vi "运维调试.vi"() -> ()   [LabVIEW 2016]
uses:
  <vilib>/Utility/miscctls.llb/LVPointTypeDef.ctl
  <vilib>/Utility/config.llb/NI_LVConfig.lvlib
panel:
  in  "运维调试菜单":T1
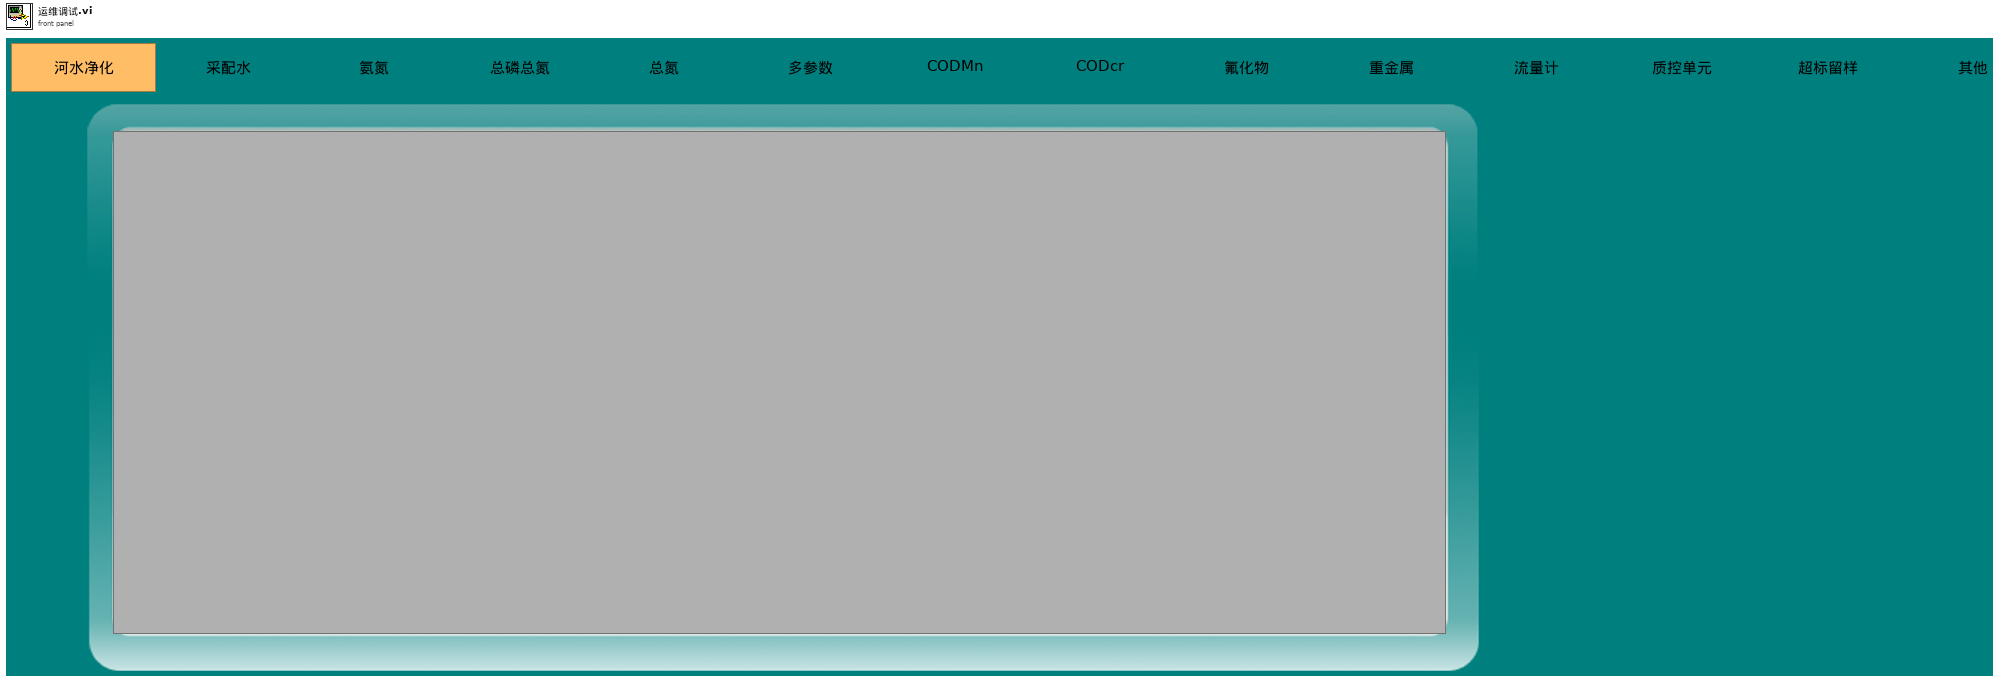
[diagram p1: front panel]
types:
  T1 = typedef "运维调试单选控件.ctl" = enum32{"河水净化", "采配水", "氨氮", "总磷总氮", "总氮", "多参数", "CODMn", "CODcr", "氟化物", "重金属", "流量计", "质控单元", "超标留样", "其他"}
  T2 = typedef "LVPointTypeDef.ctl" = cluster{"Horizontal":i16, "Vertical":i16}
  T3 = typedef "设备类型.ctl" = enum16{"微站", "固定站", "浮船"}
  T4 = typedef "采配水类型.ctl" = enum16{"V1", "V2", "V3", "V4", "室内V1", "室内V2", "固定站V1", "固定站V2", "浮船V1", "浮船V2"}
  T5 = typedef "氨氮总磷总氮模块版本.ctl" = enum16{"V2", "V3"}
  T6 = typedef "多参数模块版本.ctl" = enum16{"原位多参数", "集成式多参"}
  T7 = typedef "CODMn模块版本.ctl" = enum16{"PLC版", "单片机版", "通用流路版本"}
  T8 = typedef "CODcr模块版本.ctl" = enum16{"斯坦道V3", "点创"}
  T9 = typedef "加标回收模块版本.ctl" = enum16{"V1", "V2", "V4"}
  T10 = typedef "NI_LVConfig.lvlib/Config Data RefNum.ctl" = refnum<k1>
  T11 = enum32{"Bad", "Idle", "Run top level", "Running"}
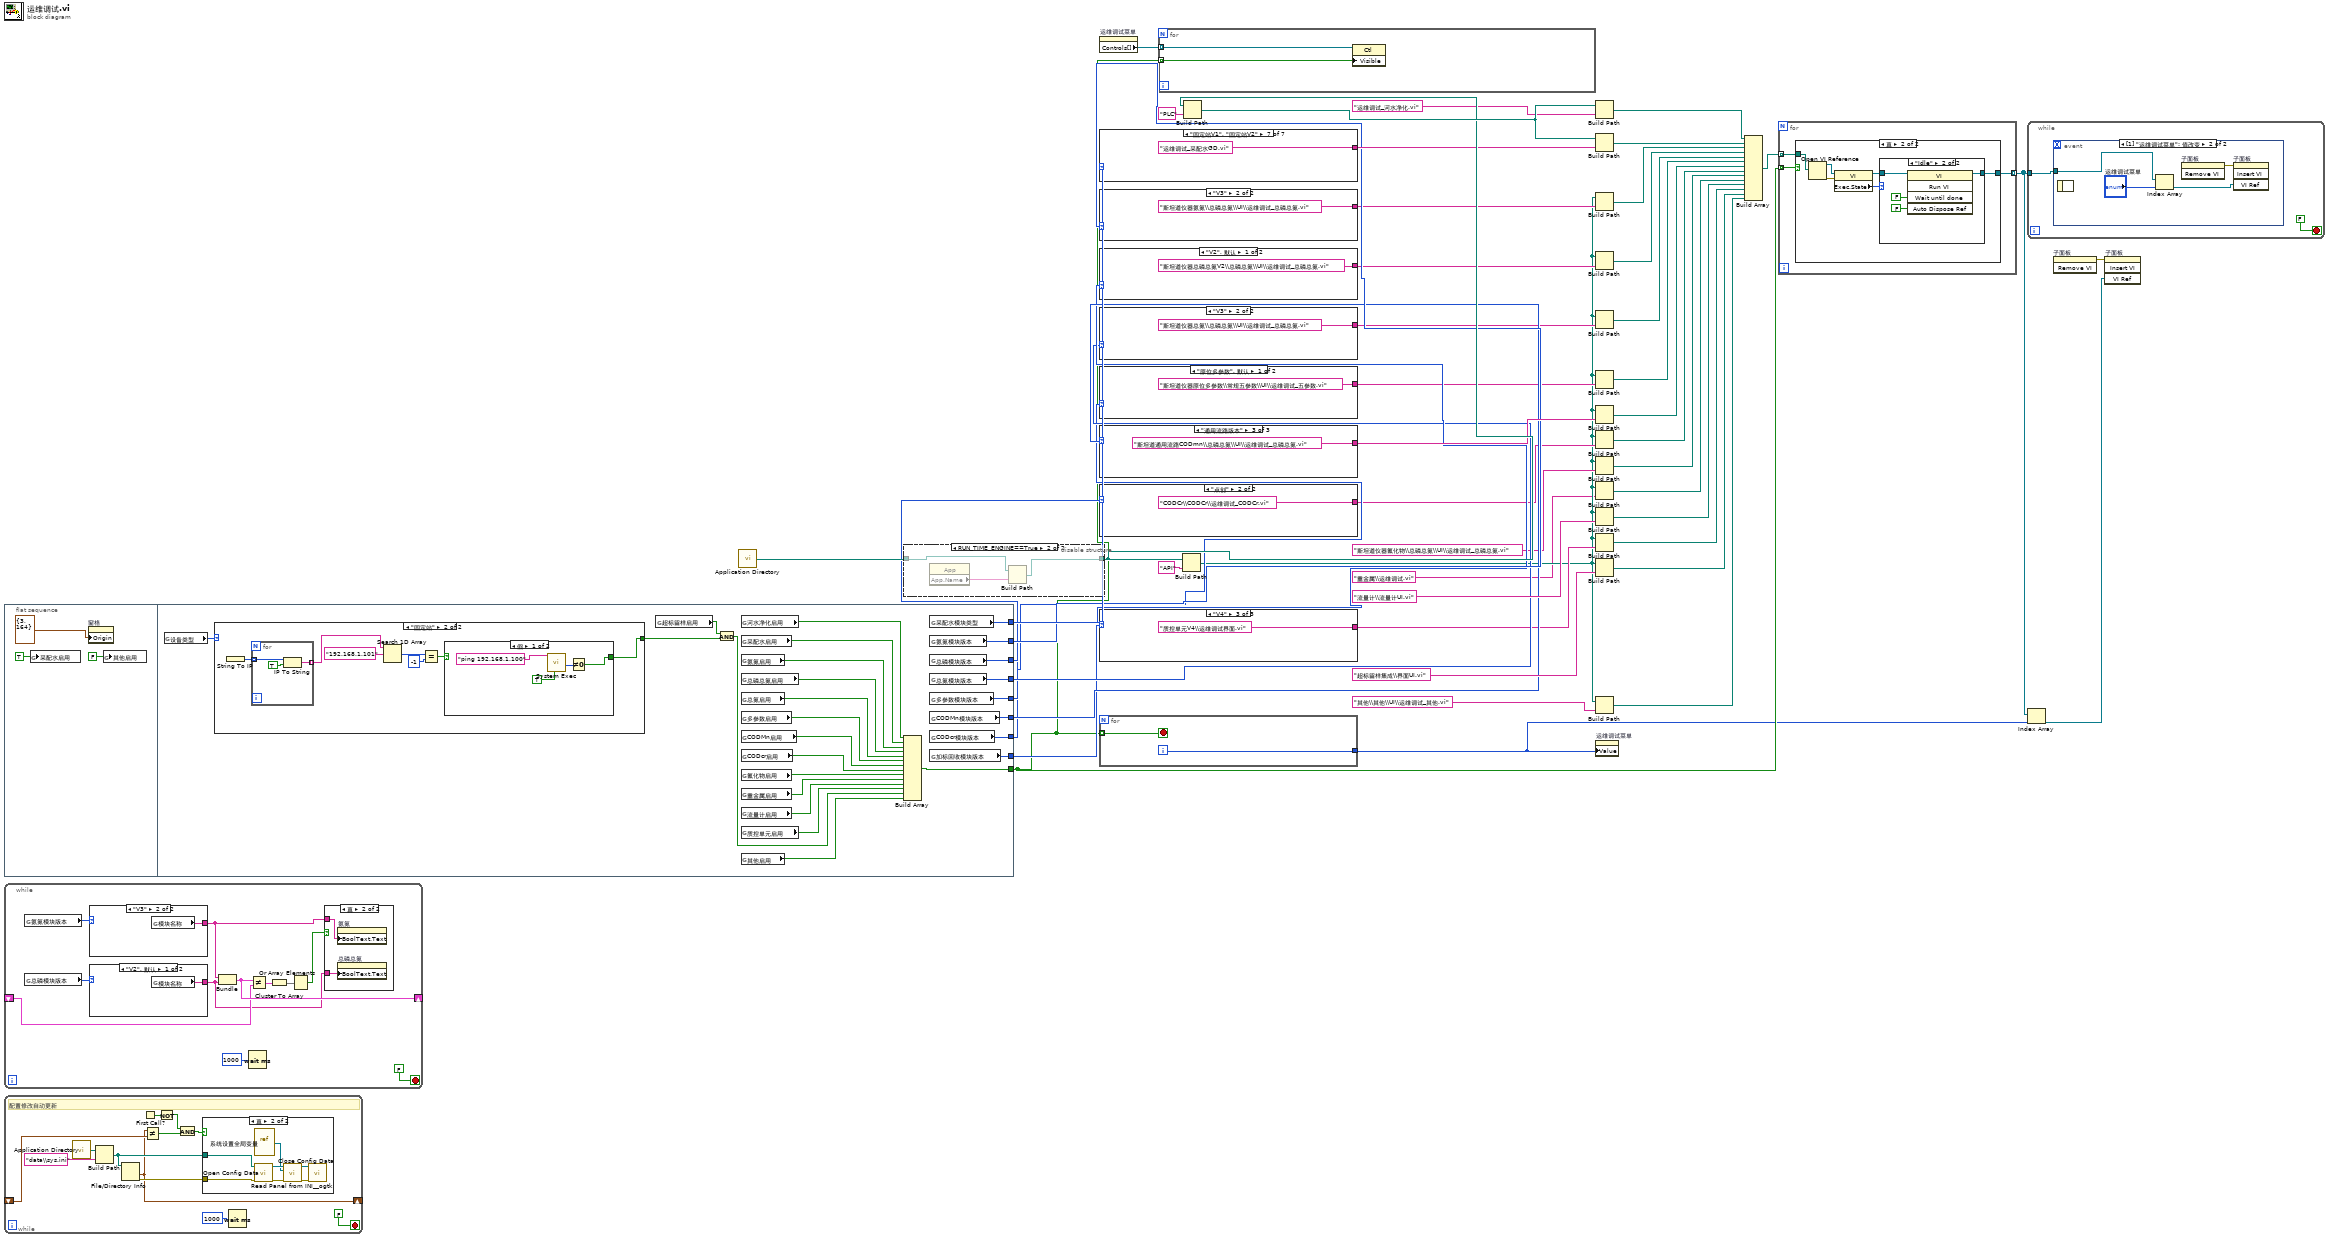
[diagram p0: block diagram]
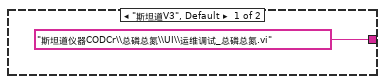
[diagram p3: hidden frame]
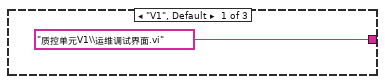
[diagram p4: hidden frame]
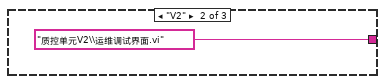
[diagram p5: hidden frame]
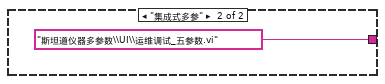
[diagram p6: hidden frame]
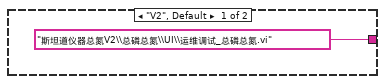
[diagram p7: hidden frame]
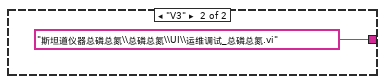
[diagram p8: hidden frame]
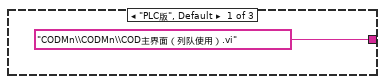
[diagram p9: hidden frame]
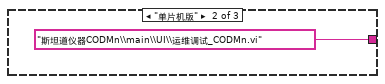
[diagram p10: hidden frame]
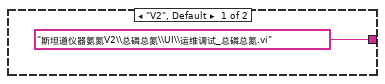
[diagram p11: hidden frame]
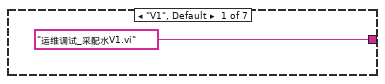
[diagram p12: hidden frame]
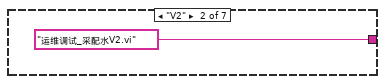
[diagram p13: hidden frame]
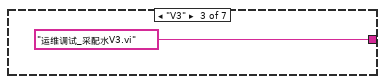
[diagram p14: hidden frame]
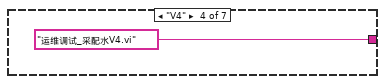
[diagram p15: hidden frame]
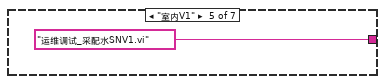
[diagram p16: hidden frame]
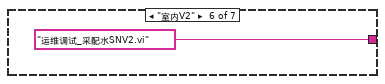
[diagram p17: hidden frame]
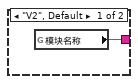
[diagram p20: hidden frame]
diagram:
  n1 = flat-sequence {
    tunnel: [w68] -> w10
    tunnel: [w65] -> w26
    tunnel: [w64] -> w25
    tunnel: [w63] -> w23
    tunnel: [w62] -> w22
    tunnel: [w61] -> w20
    tunnel: [w60] -> w18
    tunnel: [w59] -> w16
    tunnel: [w58] -> w14
    frame #0 {
      n2 = global write "系统设置全局变量.vi" "采配水启用"(TRUE ("采配水启用")) -> ()
      n3 = property on="窗格" class="Pane"("Origin"=T2 {"Horizontal"=3, "Vertical"=164} ("原点")) -> ()  [unwired: 2 in, 2 out]
      n4 = global write "系统设置全局变量.vi" "其他启用"(FALSE ("其他启用")) -> ()
    }
    frame #1 {
      n5 = global read "系统设置全局变量.vi" "设备类型"() -> (w56:T3)
      n6 = case shown="\"固定站\"" w56 {
        tunnel: [TRUE w80] -> w54
        frame "微站", Default {
        }
        frame "固定站" {
          n7 = String To IP() -> (0:w86:u32[])  [unwired: 1 in]
          n8 = for {
            tunnel: w86 -> [w94] mode=indexing
            tunnel: [w93] -> w85 mode=indexing
            n9 = IP To String(1:TRUE ("句点符号？(F)"), 2:w94) -> (0:w93:string)
          }
          n10 = Search 1D Array(1D array=w85, element="192.168.1.101" ("command line")) -> (index of element=w83:i32)  [unwired: 1 in]
          n11 = Equal?(x=w83, y=-1) -> (x = y?=w81:bool)
          n12 = case shown="假" w81 {
            tunnel: [w87 TRUE] -> w80
            frame False {
              n13 = call <vilib>:"System Exec.vi"("run minimized? (F)"=TRUE, "command line"="ping 192.168.1.100") -> ("return code"=w88:i32)  [unwired: 6 in, 3 out]
              n14 = Not Equal To 0?(x=w88) -> (x != 0?=w87:bool)
            }
            frame True {
            }
          }
        }
      }
      n15 = global read "系统设置全局变量.vi" "超标留样启用"() -> (w78:bool)
      n16 = And(x=w78, y=w54) -> (x .and. y?=w55:bool)
      n17 = global read "系统设置全局变量.vi" "河水净化启用"() -> (w69:bool)
      n18 = global read "系统设置全局变量.vi" "采配水启用"() -> (w70:bool)
      n19 = global read "系统设置全局变量.vi" "氨氮启用"() -> (w71:bool)
      n20 = global read "系统设置全局变量.vi" "总磷总氮启用"() -> (w72:bool)
      n21 = global read "系统设置全局变量.vi" "总氮启用"() -> (w66:bool)
      n22 = global read "系统设置全局变量.vi" "多参数启用"() -> (w73:bool)
      n23 = global read "系统设置全局变量.vi" "CODMn启用"() -> (w74:bool)
      n24 = global read "系统设置全局变量.vi" "CODcr启用"() -> (w75:bool)
      n25 = global read "系统设置全局变量.vi" "氟化物启用"() -> (w57:bool)
      n26 = global read "系统设置全局变量.vi" "重金属启用"() -> (w53:bool)
      n27 = global read "系统设置全局变量.vi" "流量计启用"() -> (w76:bool)
      n28 = global read "系统设置全局变量.vi" "质控单元启用"() -> (w77:bool)
      n29 = global read "系统设置全局变量.vi" "其他启用"() -> (w67:bool)
      n30 = Build Array(w69, w70, w71, w72, w66, w73, w74, w75, w57, w53, w76, w77, w55, w67) -> (w68:bool[])
      n31 = global read "系统设置全局变量.vi" "采配水模块类型"() -> (w65:T4)
      n32 = global read "系统设置全局变量.vi" "氨氮模块版本"() -> (w64:T5)
      n33 = global read "系统设置全局变量.vi" "总磷模块版本"() -> (w62:T5)
      n34 = global read "系统设置全局变量.vi" "总氮模块版本"() -> (w61:T5)
      n35 = global read "系统设置全局变量.vi" "多参数模块版本"() -> (w60:T6)
      n36 = global read "系统设置全局变量.vi" "CODMn模块版本"() -> (w63:T7)
      n37 = global read "系统设置全局变量.vi" "CODcr模块版本"() -> (w58:T8)
      n38 = global read "系统设置全局变量.vi" "加标回收模块版本"() -> (w59:T9)
    }
  }
  n39 = while {
    shift-right: [w102] -> _
    shift-left: _ -> [w101]
    stop <- FALSE stop-if-true
    n40 = global read "系统设置全局变量.vi" "氨氮模块版本"() -> (w103:T5)
    n41 = global read "系统设置全局变量.vi" "总磷模块版本"() -> (w104:T5)
    n42 = case shown="\"V3\"" w103 {
      tunnel: [w108 w109] -> w96
      frame "V2", Default {
        n43 = global read "VAR总磷总氮全局变量.vi" "模块名称"() -> (w108:string)
      }
      frame "V3" {
        n44 = global read "VAR总磷总氮全局变量.vi" "模块名称"() -> (w109:string)
      }
    }
    n45 = case shown="\"V2\", 默认" w104 {
      tunnel: [w110 w111] -> w97
      frame "V2", Default {
        n46 = global read "VAR总磷总氮全局变量.vi" "模块名称"() -> (w110:string)
      }
      frame "V3" {
        n47 = global read "VAR总磷总氮全局变量.vi" "模块名称"() -> (w111:string)
      }
    }
    n48 = Bundle("模块名称"=w96, "模块名称"=w97) -> (w102:cluster{"模块名称":string, "模块名称":string})  [unwired: 1 in]
    n49 = Wait (ms)(milliseconds to wait=u32 1000 ("等待时间（毫秒）")) -> ()  [unwired: 1 out]
    n50 = Not Equal?(x=w102, y=w101) -> (x != y?=w100:cluster{"模块名称":bool, "模块名称":bool})
    n51 = Cluster To Array(cluster=w100) -> (array=w99:bool[])
    n52 = Or Array Elements(Boolean array=w99) -> (logical OR=w98:bool)
    n53 = case shown="真" w98 {
      tunnel: w97 -> [_ w106]
      tunnel: w96 -> [_ w107]
      frame False {
      }
      frame True {
        n54 = property on="氨氮" class="Bool (严格)"("BoolText.Text"=w107) -> ()  [unwired: 2 in, 2 out]
        n55 = property on="总磷总氮" class="Bool (严格)"("BoolText.Text"=w106) -> ()  [unwired: 2 in, 2 out]
      }
    }
  }
  n56 = while {
    shift-right: [w115] -> _
    shift-left: _ -> [w118]
    stop <- FALSE stop-if-true
    # "配置修改自动更新"
    n57 = call <vilib>:"Application Directory.vi"() -> ("Application Directory"=w121:path)
    n58 = Build Path(base path=w121, name or relative path="data\\sys.ini" ("名称或相对路径")) -> (appended path=w119:path)
    n59 = File/Directory Info(path=w119) -> (last mod=w115:timestamp, error out=w116:errorcluster)  [unwired: 1 in, 5 out]
    n60 = First Call?() -> (First Call?: T/F=w113:bool)
    n61 = Not Equal?(x=w115, y=w118) -> (x != y?=w117:bool)
    n62 = Not(x=w113) -> (.not. x?=w112:bool)
    n63 = And(x=w112, y=w117) -> (x .and. y?=w114:bool)
    n64 = case shown="真" w114 {
      tunnel: w119 -> [_ w125]
      tunnel: w116 -> [_ w124]
      frame False {
      }
      frame True {
        n65 = vi-ref "系统设置全局变量.vi"() -> (w128:refnum<vi>)
        n66 = call <vilib>:"Open Config Data.vi"("error in (no error)"=w124, "configuration file path"=w125) -> ("error out"=w130:errorcluster, "refnum"=w129:T10)  [unwired: 7 in, 1 out]
        n67 = call <userlib>:"Read Panel from INI__ogtk.vi"("error in (no error)"=w130, "VI ref"=w128, "refnum"=w129) -> ("error out"=w127:errorcluster, "refnum out"=w126:T10)  [unwired: 7 in]
        n68 = call <vilib>:"Close Config Data.vi"("error in (no error)"=w127, "refnum"=w126) -> ()  [unwired: 8 in, 2 out]
      }
    }
    n69 = Wait (ms)(milliseconds to wait=u32 1000 ("等待时间（毫秒）")) -> ()  [unwired: 1 out]
  }
  n70 = call <vilib>:"Application Directory.vi"() -> ("Application Directory"=w49:path)
  n71 = disable-structure shown="RUN_TIME_ENGINE==True" {
    disable-tunnel: w49 -> [w131 w134]
    disable-tunnel: [w131 w132] -> w42
    frame condition #0 (active) {
    }
    frame condition #1 {
      n72 = property class="App"() -> ("App.Name"=w133:string)  [unwired: 2 in, 2 out]
      n73 = Build Path(base path=w134, name or relative path=w133) -> (appended path=w132:path)
    }
  }
  n74 = property on="运维调试菜单" class="RadioBtnsControl (严格)"() -> ("Controls[]"=w8:refnum<vi>[])  [unwired: 2 in, 2 out]
  n75 = case shown="\"固定站V1\", \"固定站V2\"" w26 {
    tunnel: ["运维调试_采配水V1.vi" "运维调试_采配水V2.vi" "运维调试_采配水V3.vi" "运维调试_采配水V4.vi" "运维调试_采配水SNV1.vi" "运维调试_采配水SNV2.vi" "运维调试_采配水GD.vi"] -> w27
    frame "V1", Default {
    }
    frame "V2" {
    }
    frame "V3" {
    }
    frame "V4" {
    }
    frame "室内V1" {
    }
    frame "室内V2" {
    }
    frame "固定站V1", "固定站V2" {
    }
  }
  n76 = case shown="\"V3\"" w25 {
    tunnel: ["斯坦道仪器氨氮V2\\总磷总氮\\UI\\运维调试_总磷总氮.vi" ("名称或相对路径") "斯坦道仪器氨氮\\总磷总氮\\UI\\运维调试_总磷总氮.vi" ("名称或相对路径")] -> w24
    frame "V2", Default {
    }
    frame "V3" {
    }
  }
  n77 = case shown="\"V2\", 默认" w22 {
    tunnel: ["斯坦道仪器总磷总氮V2\\总磷总氮\\UI\\运维调试_总磷总氮.vi" ("名称或相对路径") "斯坦道仪器总磷总氮\\总磷总氮\\UI\\运维调试_总磷总氮.vi" ("名称或相对路径")] -> w21
    frame "V2", Default {
    }
    frame "V3" {
    }
  }
  n78 = case shown="\"V3\"" w20 {
    tunnel: ["斯坦道仪器总氮V2\\总磷总氮\\UI\\运维调试_总磷总氮.vi" ("名称或相对路径") "斯坦道仪器总氮\\总磷总氮\\UI\\运维调试_总磷总氮.vi" ("名称或相对路径")] -> w19
    frame "V2", Default {
    }
    frame "V3" {
    }
  }
  n79 = case shown="\"原位多参数\", 默认" w18 {
    tunnel: ["斯坦道仪器原位多参数\\常规五参数\\UI\\运维调试_五参数.vi" ("名称或相对路径") "斯坦道仪器多参数\\UI\\运维调试_五参数.vi" ("名称或相对路径")] -> w17
    frame "原位多参数", Default {
    }
    frame "集成式多参" {
    }
  }
  n80 = case shown="\"通用流路版本\"" w23 {
    tunnel: ["CODMn\\CODMn\\COD主界面（列队使用）.vi" ("名称或相对路径") "斯坦道仪器CODMn\\main\\UI\\运维调试_CODMn.vi" ("名称或相对路径") "斯坦道通用流路CODmn\\总磷总氮\\UI\\运维调试_总磷总氮.vi" ("名称或相对路径")] -> w29
    frame "PLC版", Default {
    }
    frame "单片机版" {
    }
    frame "通用流路版本" {
    }
  }
  n81 = case shown="\"点创\"" w14 {
    tunnel: ["斯坦道仪器CODCr\\总磷总氮\\UI\\运维调试_总磷总氮.vi" ("名称或相对路径") "CODCr\\CODCr\\运维调试_CODCr.vi" ("名称或相对路径")] -> w13
    frame "斯坦道V3", Default {
    }
    frame "点创" {
    }
  }
  n82 = case shown="\"V4\"" w16 {
    tunnel: ["质控单元V1\\运维调试界面.vi" ("名称或相对路径") "质控单元V2\\运维调试界面.vi" ("名称或相对路径") "质控单元V4\\运维调试界面.vi" ("名称或相对路径")] -> w15
    frame "V1", Default {
    }
    frame "V2" {
    }
    frame "V4" {
    }
  }
  n83 = for {
    tunnel: w10 -> [w159] mode=indexing
    tunnel: [w158] -> w5
    i -> [w158]
    stop <- w159 stop-if-true
  }
  n84 = for {
    tunnel: w10 -> [w160] mode=indexing
    tunnel: w8 -> [w161] mode=indexing
    n85 = property class="Ctl"(reference=w161, "Visible"=w160) -> ()  [unwired: 1 in, 2 out]
  }
  n86 = Build Path(base path=w42, name or relative path="API" ("名称或相对路径")) -> (appended path=w3:path)
  n87 = Build Path(base path=w42, name or relative path="PLC" ("名称或相对路径")) -> (appended path=w44:path)
  n88 = Build Path(base path=w44, name or relative path="运维调试_河水净化.vi" ("名称或相对路径")) -> (appended path=w32:path)
  n89 = Build Path(base path=w44, name or relative path=w27) -> (appended path=w31:path)
  n90 = Build Path(base path=w3, name or relative path=w24) -> (appended path=w41:path)
  n91 = Build Path(base path=w3, name or relative path=w21) -> (appended path=w40:path)
  n92 = Build Path(base path=w3, name or relative path=w19) -> (appended path=w39:path)
  n93 = Build Path(base path=w3, name or relative path=w17) -> (appended path=w38:path)
  n94 = Build Path(base path=w3, name or relative path=w29) -> (appended path=w37:path)
  n95 = Build Path(base path=w3, name or relative path=w13) -> (appended path=w36:path)
  n96 = Build Path(base path=w3, name or relative path="斯坦道仪器氟化物\\总磷总氮\\UI\\运维调试_总磷总氮.vi" ("名称或相对路径")) -> (appended path=w11:path)
  n97 = Build Path(base path=w3, name or relative path="重金属\\运维调试.vi" ("名称或相对路径")) -> (appended path=w1:path)
  n98 = Build Path(base path=w3, name or relative path="流量计\\流量计UI.vi" ("名称或相对路径")) -> (appended path=w4:path)
  n99 = Build Path(base path=w3, name or relative path=w15) -> (appended path=w35:path)
  n100 = Build Path(base path=w3, name or relative path="超标留样集成\\界面UI.vi" ("名称或相对路径")) -> (appended path=w34:path)
  n101 = Build Path(base path=w3, name or relative path="其他\\其他\\UI\\运维调试_其他.vi" ("名称或相对路径")) -> (appended path=w33:path)
  n102 = property on="运维调试菜单" class="RadioBtnsControl (严格)"("Value"=w5) -> ()  [unwired: 2 in, 2 out]
  n103 = Build Array(w32, w31, w41, w40, w39, w38, w37, w36, w11, w1, w4, w35, w34, w33) -> (w30:path[])
  n104 = for {
    tunnel: w30 -> [w164] mode=indexing
    tunnel: [w163] -> w9 mode=indexing
    tunnel: w10 -> [w162] mode=indexing
    n105 = case shown="真" w162 {
      tunnel: w164 -> [_ w169]
      tunnel: [_ w166] -> w163
      frame False {
      }
      frame True {
        n106 = Open VI Reference(vi path=w169) -> (vi reference=w168:refnum<vi>, error out=w167:errorcluster)  [unwired: 5 in]
        n107 = property class="VI"(reference=w168, error in=w167) -> (reference out=w165:refnum<vi>, "Exec.State"=w170:T11)  [unwired: 1 out]
        n108 = case shown="\"Idle\"" w170 {
          tunnel: w165 -> [w171 w173]
          tunnel: [w171 w172] -> w166
          frame "Bad", Default {
          }
          frame "Idle" {
            n109 = invoke class="VI" method="Run VI"(reference=w173, "Wait until done"=FALSE ("结束前等待"), "Auto Dispose Ref"=FALSE ("自动销毁引用")) -> (reference out=w172:refnum<vi>)  [unwired: 2 in, 4 out]
          }
        }
      }
    }
  }
  n110 = while {
    tunnel: w9 -> [w176]
    stop <- FALSE stop-if-true
    n111 = event shown="[1] \"运维调试菜单\": 值改变" {
      selector: _ -> [_ _]
      dyn-events: _ -> [_ _]
      timeout: _ -> [_ _]
      tunnel: w176 -> [_ w178]
      event Timeout {
        n112 = event-data() -> ()  [unwired: 1 in, 3 out]
      }
      event Value Change {
        n113 = event-data() -> ()  [unwired: 1 in, 1 out]
        n114 = Index Array(array=w178, index="运维调试菜单") -> (element=w180:refnum<vi>)
        n115 = invoke on="子面板" class="SubPnl" method="Remove VI"() -> (error out=w181:errorcluster)  [unwired: 3 in, 2 out]
        n116 = invoke on="子面板" class="SubPnl" method="Insert VI"(error in=w181, "VI Ref"=w180) -> ()  [unwired: 2 in, 4 out]
      }
    }
  }
  n117 = Index Array(array=w9, index=w5) -> (element=w7:refnum<vi>)
  n118 = invoke on="子面板" class="SubPnl" method="Remove VI"() -> (error out=w6:errorcluster)  [unwired: 3 in, 2 out]
  n119 = invoke on="子面板" class="SubPnl" method="Insert VI"(error in=w6, "VI Ref"=w7) -> ()  [unwired: 2 in, 4 out]
